vi "Arduino_comms_Global.vi"() -> ()   [LabVIEW 2014]
uses:
  ADAM Serial/Instrument drivers/Arduino/ctls_and_globals/Arduino Config & resource typedef.ctl
panel:
  in  "Arduino VISA config & resource":T1[](array[typedef])=[{"VISA resource name"="COM15", "baud rate (bps)"=115200, "timeout (ms)"=1000, "data bits"=8, "parity"=enum."None", "stop bits (10: 1 bit)"=10, "flow control"=0, "termination char (hex)"=10, "Enable Termination Char"=TRUE, "byte count"=64, "Resource locked?"=FALSE}, {"VISA resource name"="COM23", "baud rate (bps)"=115200, "timeout (ms)"=1000, "data bits"=8, "parity"=enum."None", "stop bits (10: 1 bit)"=10, "flow control"=0, "termination char (hex)"=10, "Enable Termination Char"=FALSE, "byte count"=4, "Resource locked?"=FALSE}] {"termination char (hex)" format="%02x"; "stop bits (10: 1 bit)" items=["1.0"=10, "1.5"=15, "2.0"=20]; "flow control" items=["None", "XON/XOFF", "RTS/CTS", "XON/XOFF & RTS/CTS", "DTR/DSR", "XON/XOFF & DTR/DSR"]}
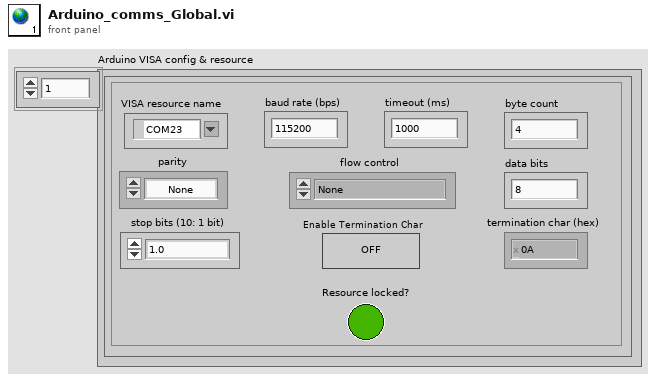
[diagram p1: front panel]
types:
  T1 = typedef "Arduino Config & resource typedef.ctl" = cluster{"VISA resource name":refnum<visa-resource-name>, "baud rate (bps)":u32, "timeout (ms)":u32, "data bits":u16, "parity":enum16{"None", "Odd", "Even", "Mark", "Space"}, "stop bits (10: 1 bit)":u16, "flow control":u16, "termination char (hex)":u8, "Enable Termination Char":bool, "byte count":u32, "Resource locked?":bool}
diagram:
